vi "PLC_CODMn 获取仪器状态.vi"() -> (3 "CODMn状态":u16(ring) caption="氨氮状态" items=["待机", "润洗", "进样", "进样完成", "柱塞泵加标", "等待取液", "排液"])   [LabVIEW 2016, in "质控单元V4.lvlib"]
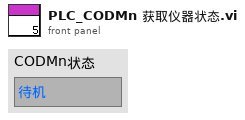
[diagram p1: front panel]
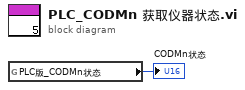
[diagram p0: block diagram]
diagram:
  n1 = global read "系统交互.vi" "PLC版_CODMn状态"() -> (→"CODMn状态":u16)
